vi "Logger-Add.vi"(8 "error in":errorcluster, 11 "HandledFileContent":T1 {"Values" format="%.3f"}) -> (0 "error out":errorcluster)   [LabVIEW 2016]
uses:
  Logger.FileBody.ctl
  Logger.Action.ctl
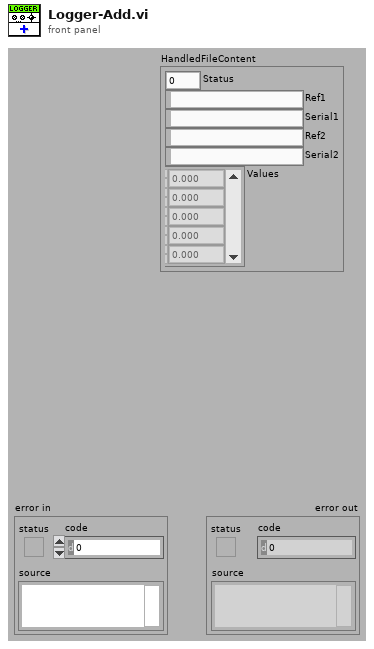
[diagram p1: front panel]
types:
  T1 = typedef "Logger.FileBody.ctl" = cluster{"Status":u8, "Ref1":string, "Serial1":string, "Ref2":string, "Serial2":string, "Values":sgl[]}
  T2 = typedef "Logger.Action.ctl" = enum32{"idle", "constructor", "destructor", "--- Logger ---", "Begin", "Add", "End"}
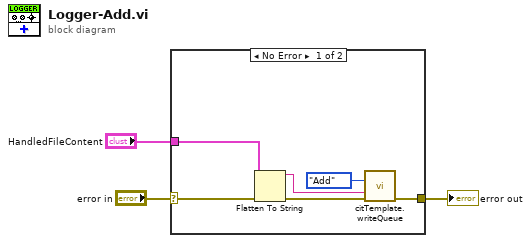
[diagram p0: block diagram]
diagram:
  n1 = case shown="No Error" "error in" {
    selector: "error in" -> [w8 w10]
    tunnel: [w9 w10] -> w2
    tunnel: "HandledFileContent" -> [w4 _]
    frame No Error {
      n2 = Flatten To String(anything=w4, error in (no error)=w8) -> (data string=w6:string, error out=w7:errorcluster)  [unwired: 2 in, 1 out]
      n3 = call "citTemplate.writeQueue.vi"("event in (if not connected:all statemachine with data event)"=Logger.Action."Add" ("Action"), "data in"=w6, "error in (no error)"=w7) -> ("error out"=w9:errorcluster)  [unwired: 12 in]
    }
    frame Error {
    }
  }
  "error out" <- w2
